vi "visa_write+crlf.vi"(8 "error in (no error)":errorcluster, 10 "Strings (empty)":string, 11 "VISA resource name":refnum<visa-resource-name>) -> (0 "error out":errorcluster, 3 "VISA resource name out":refnum<visa-resource-name>)   [LabVIEW 2021, in "Ceyear.lvlib"]
uses:
  <instrlib>/Ceyear/Ceyear.lvlib
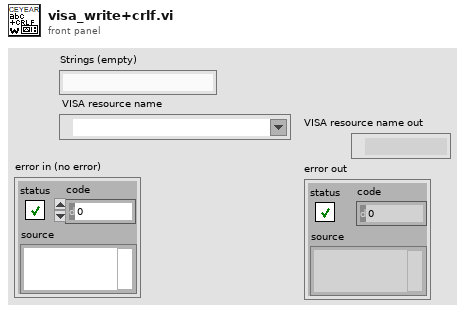
[diagram p1: front panel]
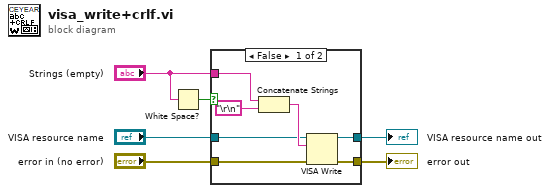
[diagram p0: block diagram]
diagram:
  n1 = White Space?(1:"Strings (empty)") -> (0:w2:bool)
  n2 = case shown="False" w2 {
    tunnel: "VISA resource name" -> [w11 w15]
    tunnel: [w10 w15] -> w5
    tunnel: "Strings (empty)" -> [w9 _]
    tunnel: "error in (no error)" -> [w8 w14]
    tunnel: [w7 w14] -> w3
    frame False {
      n3 = Concatenate Strings(w9, "\r\n") -> (w12:string)
      n4 = VISA Write(VISA resource name=w11, write buffer=w12, error in (no error)=w8) -> (VISA resource name out=w10:refnum<visa-resource-name>, error out=w7:errorcluster)  [unwired: 1 out]
    }
    frame True {
    }
  }
  "VISA resource name out" <- w5
  "error out" <- w3
